vi "n！.vi"() -> ()   [LabVIEW 2009]
panel:
  out "n!":dbl
  in  "求n！，n=？":i32
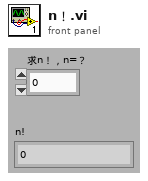
[diagram p1: front panel]
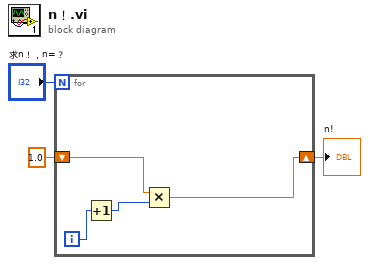
[diagram p0: block diagram]
diagram:
  n1 = for {
    N: "求n！，n=？" -> [_]
    shift-right: [w7] -> w1
    shift-left: 1.0 -> [w4]
    i -> [w6]
    n2 = Increment(x=w6) -> (x+1=w5:i32)
    n3 = Multiply(x=w4, y=w5) -> (x*y=w7:dbl)
  }
  "n!" <- w1
